vi "BugReportURL.vi"() -> (1 "BugReportURL":string)   [LabVIEW 2020]
doc: "*-----------------------------------------------------\n* Author: SWatts\n*\n* VI Description: VI Constant that contains the URL to the bug report system for this application, can be updated by Deploy if required\n* \n*\n* Error handling: All errors passed out\n*\n* Pre-condition: \n*\n* Post-condition: None\n*\n* Revision History:\n*\n* Rev Date Author Description \n* 01 30/04/2014 SWatts First issue\n*\n*-----------------------------------------------------"
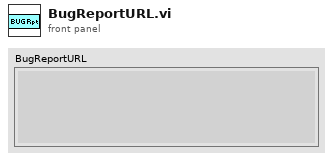
[diagram p1: front panel]
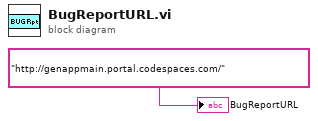
[diagram p0: block diagram]
diagram:
  "BugReportURL" <- "http://genappmain.portal.codespaces.com/" ("Link")
